vi "Clean Up After Init Error.vi"(6 "session initialization parameters":T1, 7 "remote connection options":T2, 8 "error in":errorcluster, 9 "initialize and close session behavior":T3, 10 "session in":variant, 11 "session factory in":refnum<class "ISession Factory.lvclass">) -> (0 "error out":errorcluster)   [LabVIEW 2020, in "MeasurementLink Instrument.lvlib" / "ISession Factory.lvclass"]
doc: "Closes the local session in the event that an error occurred while creating a set of sessions. If the session represents a remote session, <b>initialize and close session behavior</b> indicates whether the remote session was created or attached to when initializing the local session. The default implementation sends \"Create and Close\" or \"Attach and Detach\" respectively to the \"Close MeasurementLink Session\" VI."
uses:
  ISession Factory.lvclass
  Initialize and Close Session Behavior.ctl
  Remote Connection Options.ctl
  Session Initialization Parameters.ctl
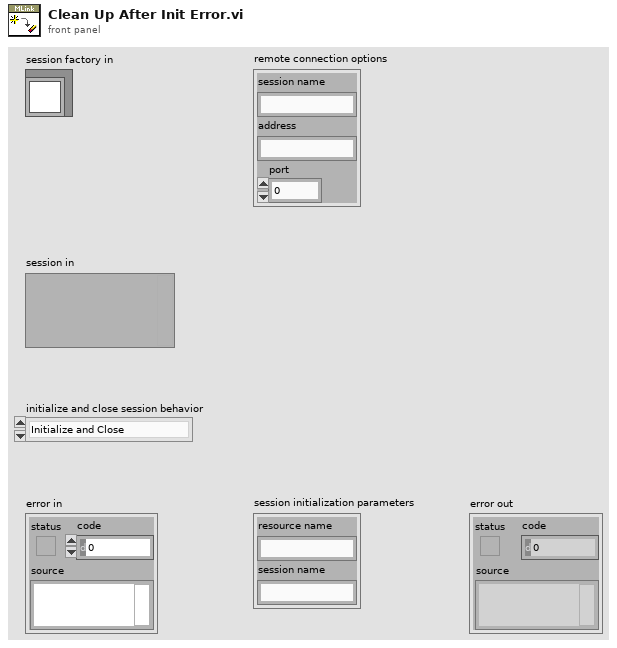
[diagram p1: front panel]
types:
  T1 = typedef "MeasurementLink Instrument.lvlib/ISession Factory.lvclass/Session Initialization Parameters.ctl" = cluster{"resource name":string, "session name":string}
  T2 = typedef "MeasurementLink Instrument.lvlib/ISession Factory.lvclass/Remote Connection Options.ctl" = cluster{"session name":string, "address":string, "port":u32}
  T3 = typedef "MeasurementLink Instrument.lvlib/ISession Factory.lvclass/Initialize and Close Session Behavior.ctl" = enum16{"Initialize and Close", "Attach and Detach", "Initialize and Detach", "Attach and Close"}
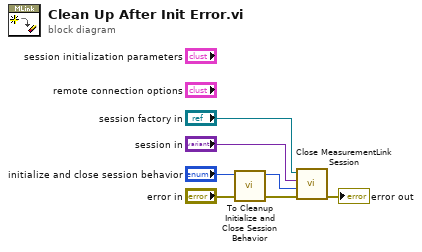
[diagram p0: block diagram]
diagram:
  n1 = call "To Cleanup Initialize and Close Session Behavior.vi"("initialize and close session behavior"="initialize and close session behavior") -> ("cleanup initialize and close session behavior"=w1:T3)  [unwired: 10 in]
  n2 = call-dynamic "Close MeasurementLink Session.vi"("error in (no error)"="error in", "initialize and close session behavior"=w1, "session in"="session in", "session factory in"="session factory in") -> ("error out"=→"error out":errorcluster)  [unwired: 7 in]
